vi "Get Underline.vi"(8 "error in (no error)":errorcluster, 11 "Style in":refnum<class "Style.lvclass">) -> (0 "error out":errorcluster, 2 "Underline":T1=18 items=["Single"=1, "Words"=2, "Double"=3, "Thick"=4, "Dotted"=5, "DottedHeavy"=6, "Dash"=7, "DashedHeavy"=8, "DashLong"=9, "DashLongHeavy"=10, "DotDash"=11, "DashDotHeavy"=12, "DotDotDash"=13, "DashDotDotHeavy"=14, "Wave"=15, "WavyHeavy"=16, "WavyDouble"=17, "None"=18], 3 "Style out":refnum<class "Style.lvclass">)   [LabVIEW 2017, in "Styles.lvlib" / "Style.lvclass"]
uses:
  Style.lvclass
  Underline--ring.ctl
  Style.lvclass/Style.ctl
  Styles.lvlib
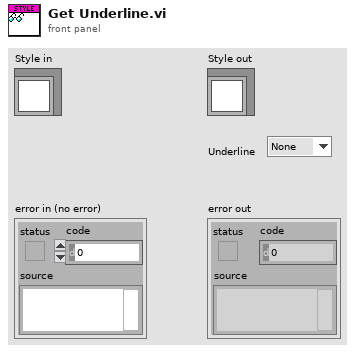
[diagram p1: front panel]
types:
  T1 = typedef "Styles.lvlib/Underline--ring.ctl" = i32
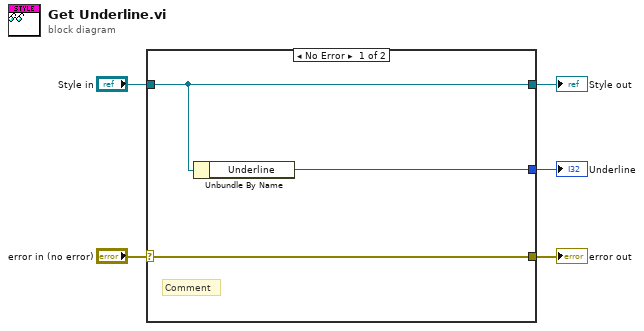
[diagram p0: block diagram]
diagram:
  n1 = case shown="No Error" "error in (no error)" {
    selector: "error in (no error)" -> [w8 w9]
    tunnel: [w8 w9] -> w4
    tunnel: [w7 w10] -> w2
    tunnel: "Style in" -> [w7 w10]
    tunnel: [w6 _] -> w1
    frame No Error {
      # "Comment"
      n2 = Unbundle By Name(w7) -> ("Underline"=w6:T1)
    }
    frame Error {
    }
  }
  "error out" <- w4
  "Style out" <- w2
  "Underline" <- w1
